vi "Set Drive Motors.vi"(5 "Disable":bool, 6 "Drive PID Slot":i32, 7 "Max Velocity(CP100ms)":dbl=200.0, 8 "Control Mode":T1 items=["PercentOutput"=0, "Position"=1, "Velocity"=2, "Current"=3, "Follower"=5, "MotionProfile"=6, "MotionMagic"=7, "MotionProfileArc"=10, "Disabled"=15], 9 "Motor List":T2[](array[typedef])=[enum."Right-Front", enum."Left-Front", enum."Left-Back", enum."Right-Back"], 10 "Swerve Data":T3 {"Back Right"."Angle" scale format="%.3f"; "Back Right"."Velocity" scale=-1.0..1.0 scale format="%.1f"; "Back Left"."Angle" scale format="%.3f"; "Back Left"."Velocity" scale=-1.0..1.0 scale format="%.1f"; "Front Left"."Angle" scale format="%.3f"; "Front Left"."Velocity" scale=-1.0..1.0 scale format="%.1f"; "Front Right"."Angle" scale format="%.3f"; "Front Right"."Velocity" scale=-1.0..1.0 scale format="%.1f"}, 11 "Drive Refs":T7[](array[typedef])) -> (1 "Speeds":dbl[](array[numeric]), 3 "Array Out":T7[](array[typedef]))   [LabVIEW 2023, in "Thor-SwerveDrive_ACT.lvlib"]
uses:
  Thor-SwerveDrive_ACT.lvlib
  <vilib>/Rock Robotics/WPI/ThirdParty/Phoenix-LabVIEW/Motor Controller/Controls/CTRE_Phoenix_MotorControl_ControlMode.ctl
  <vilib>/Rock Robotics/SystemInterfaces/DIO/FPGA_DIOPWMChannel.ctl
  <vilib>/Rock Robotics/WPI/PWM/WPI_PWMDeadband.ctl
  <vilib>/Rock Robotics/WPI/MotorControl/WPI_MotorControlType.ctl
  <vilib>/Rock Robotics/SystemInterfaces/DIO/FPGA_DIOChannel.ctl
  <vilib>/Rock Robotics/WPI/MotorControl/WPI_MotorControlDeviceRef.ctl
  Shared Code/TypeDefs/Level_Velocity plus-minus 1.ctl
  Shared Code/TypeDefs/Dial_Compase heading unit circle CCW positive.ctl
  Shared Code/TypeDefs/Cluster_Module Velocity-Direction-Rotations.ctl
  Shared Code/TypeDefs/Cluster_Swerve 4 Steer and Velocity.ctl
  Shared Code/TypeDefs/ENUM_Motor Index.ctl
panel:
  # "\"Front\" of Robot"
  # "Right Hand Rule"
  # "X"
  # "+CCW"
  # "Y"
  # "(0,0)"
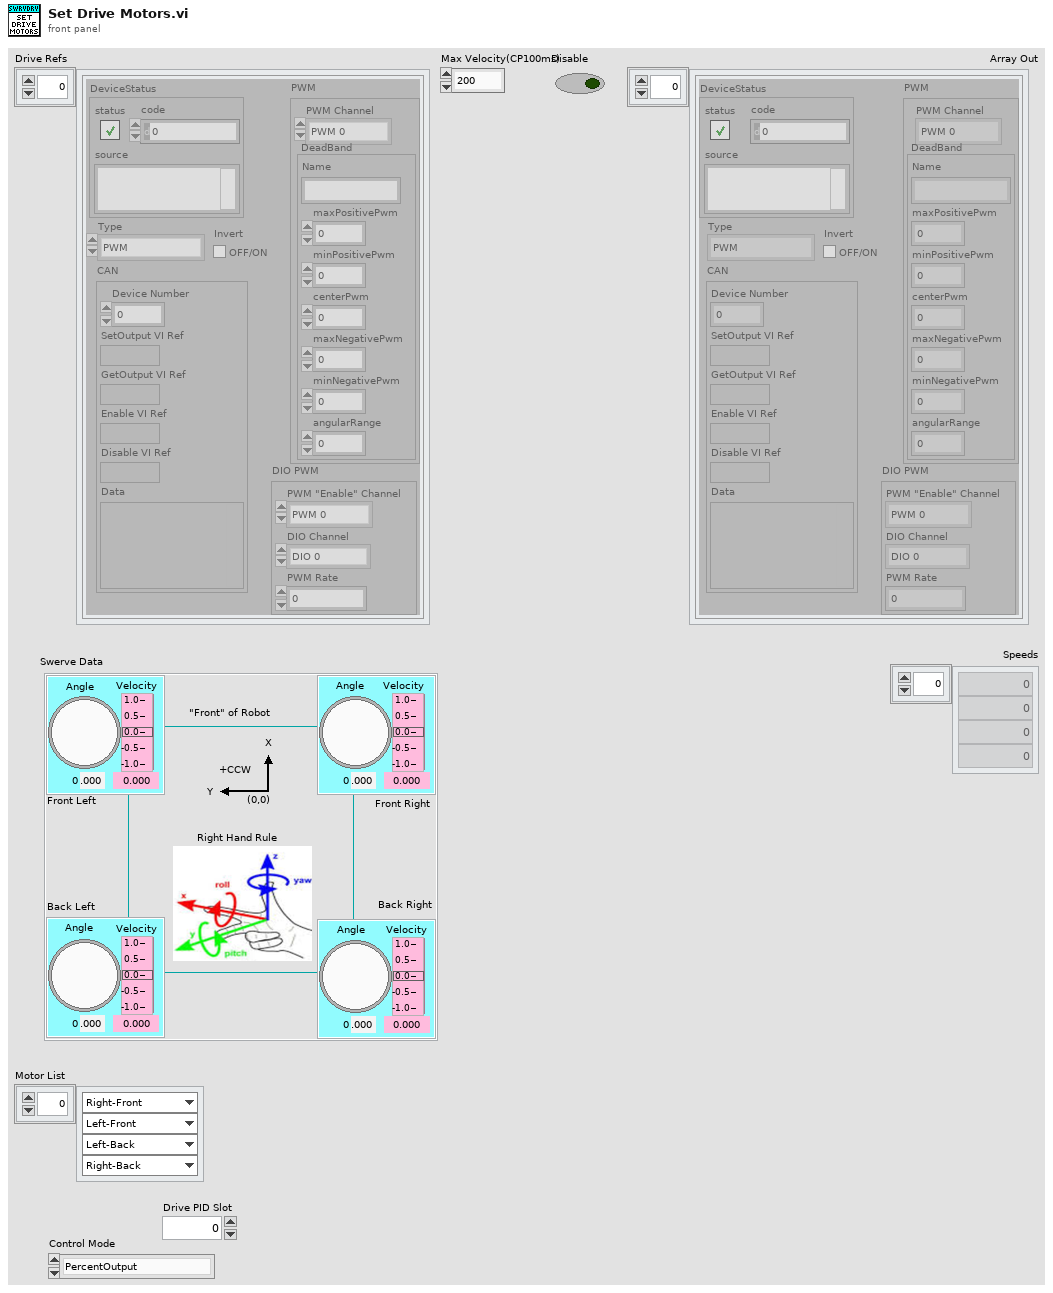
[diagram p1: front panel]
types:
  T1 = typedef "CTRE_Phoenix_MotorControl_ControlMode.ctl" = u16
  T2 = typedef "ENUM_Motor Index.ctl" = enum16{"Left-Front", "Right-Front", "Left-Back", "Right-Back"}
  T3 = typedef "Cluster_Swerve 4 Steer and Velocity.ctl" = cluster{"Front Right":T4, "Front Left":T4, "Back Left":T4, "Back Right":T4}
  T4 = typedef "Cluster_Module Velocity-Direction-Rotations.ctl" = cluster{"Velocity":T5, "Angle":T6, "Rotations Count":dbl}
  T5 = typedef "Level_Velocity plus-minus 1.ctl" = dbl
  T6 = typedef "Dial_Compase heading unit circle CCW positive.ctl" = dbl
  T7 = typedef "WPI_MotorControlDeviceRef.ctl" = cluster{"DeviceStatus":errorcluster, "Type":T8, "PWM":cluster{"PWM Channel":T9, "DeadBand":T10}, "CAN":cluster{"Device Number":u8, "SetOutput VI Ref":variant, "GetOutput VI Ref":variant, "Enable VI Ref":variant, "Disable VI Ref":variant, "Data":variant}, "Invert":bool, "DIO PWM":cluster{"PWM \"Enable\" Channel":T9, "DIOChannel":T11, "PWM Rate":dbl}}
  T8 = typedef "WPI_MotorControlType.ctl" = enum16{"PWM", "CAN", "DIO PWM"}
  T9 = typedef "FPGA_DIOPWMChannel.ctl" = enum8{"PWM 0", "PWM 1", "PWM 2", "PWM 3", "PWM 4", "PWM 5", "PWM 6", "PWM 7", "PWM 8", "PWM 9", "PWM MXP 0", "PWM MXP 1", "PWM MXP 2", "PWM MXP 3", "PWM MXP 4", "PWM MXP 5", "PWM MXP 6", "PWM MXP 7", "PWM MXP 8", "PWM MXP 9", "Invalid"}
  T10 = typedef "WPI_PWMDeadband.ctl" = cluster{"Name":string, "maxPositivePwm":i32, "minPositivePwm":i32, "centerPwm":i32, "maxNegativePwm":i32, "minNegativePwm":i32, "angularRange":u16}
  T11 = typedef "FPGA_DIOChannel.ctl" = enum8{"DIO 0", "DIO 1", "DIO 2", "DIO 3", "DIO 4", "DIO 5", "DIO 6", "DIO 7", "DIO 8", "DIO 9", "DIO MXP 0", "DIO MXP 1", "DIO MXP 2", "DIO MXP 3", "DIO MXP 4", "DIO MXP 5", "DIO MXP 6", "DIO MXP 7", "DIO MXP 8", "DIO MXP 9", "DIO MXP 10", "DIO MXP 11", "DIO MXP 12", "DIO MXP 13", "DIO MXP 14", "DIO MXP 15", "SPI Port CS1", "SPI Port CS2", "SPI Port CS3", "SPI Port MISO", "SPI Port MOSI", "Invalid"}
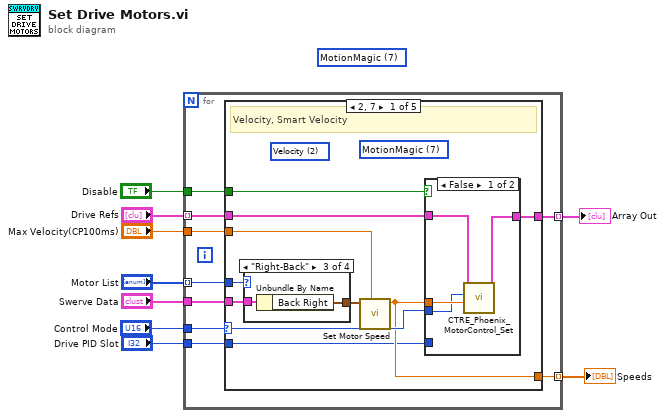
[diagram p0: block diagram]
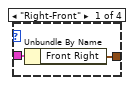
[diagram p3: hidden frame]
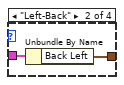
[diagram p4: hidden frame]
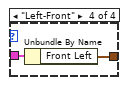
[diagram p5: hidden frame]
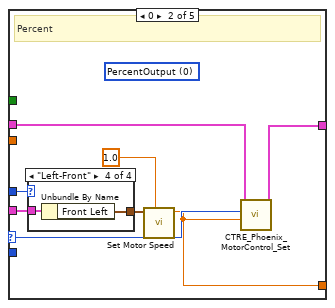
[diagram p6: hidden frame]
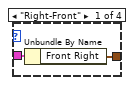
[diagram p7: hidden frame]
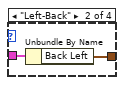
[diagram p8: hidden frame]
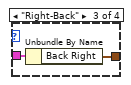
[diagram p9: hidden frame]
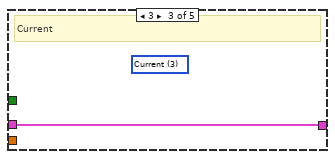
[diagram p10: hidden frame]
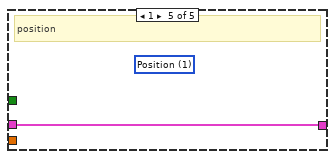
[diagram p12: hidden frame]
diagram:
  (unwired) T1 7 items=["PercentOutput"=0, "Position"=1, "Velocity"=2, "Current"=3, "Follower"=5, "MotionProfile"=6, "MotionMagic"=7, "MotionProfileArc"=10, "Disabled"=15] ("Control Mode")
  n1 = for {
    tunnel: "Drive Refs" -> [w18] mode=indexing
    tunnel: "Control Mode" -> [w17]
    tunnel: "Drive PID Slot" -> [w16]
    tunnel: [w15] -> w9 mode=indexing
    tunnel: "Max Velocity(CP100ms)" -> [w12]
    tunnel: "Motor List" -> [w14] mode=indexing
    tunnel: "Swerve Data" -> [w13]
    tunnel: [w11] -> w3 mode=indexing
    tunnel: "Disable" -> [w10]
    n2 = case shown="2, 7" w17 {
      selector: w17 -> [w27 w48 _ _ _]
      tunnel: w18 -> [w28 w49 w58 w59 w60]
      tunnel: w16 -> [w20 _ _ _ _]
      tunnel: [w26 w47 w58 w59 w60] -> w15
      tunnel: w14 -> [w24 w45 _ _ _]
      tunnel: w13 -> [w25 w46 _ _ _]
      tunnel: w12 -> [w22 _ _ _ _]
      tunnel: [w21 w42 _ _ _] -> w11
      tunnel: w10 -> [w19 _ _ _ _]
      frame 2, 7 {
        (unwired) T1 7 items=["PercentOutput"=0, "Position"=1, "Velocity"=2, "Current"=3, "Follower"=5, "MotionProfile"=6, "MotionMagic"=7, "MotionProfileArc"=10, "Disabled"=15] ("Control Mode")
        (unwired) T1 2 items=["PercentOutput"=0, "Position"=1, "Velocity"=2, "Current"=3, "Follower"=5, "MotionProfile"=6, "MotionMagic"=7, "MotionProfileArc"=10, "Disabled"=15] ("Control Mode")
        # "Velocity, Smart Velocity"
        n3 = case shown="\"Right-Back\"" w24 {
          tunnel: w25 -> [w35 w37 w39 w41]
          tunnel: [w34 w36 w38 w40] -> w23
          frame "Right-Front" {
            n4 = Unbundle By Name(w35) -> ("Front Right"=w34:T4)
          }
          frame "Left-Back" {
            n5 = Unbundle By Name(w37) -> ("Back Left"=w36:T4)
          }
          frame "Right-Back" {
            n6 = Unbundle By Name(w39) -> ("Back Right"=w38:T4)
          }
          frame "Left-Front" {
            n7 = Unbundle By Name(w41) -> ("Front Left"=w40:T4)
          }
        }
        n8 = call "Set Motor Speed.vi"("Max Velocity"=w22, "Front Left"=w23) -> ("Velocity Value Set Out"=w21:dbl)  [unwired: 9 in]
        n9 = case shown="False" w19 {
          tunnel: w28 -> [w32 w33]
          tunnel: w27 -> [w29 _]
          tunnel: [w31 w33] -> w26
          tunnel: w21 -> [w30 _]
          tunnel: w20 -> [_ _]
          frame False {
            n10 = call <vilib>:"CTRE_Phoenix_MotorControl_Set.vi"("Output"=w30, "Control Mode"=w29, "PhoenixMotorControlDevRef"=w32) -> ("PhoenixMotorControlDevRef"=w31:T7)  [unwired: 7 in, 1 out]
          }
          frame True {
          }
        }
      }
      frame 0 {
        (unwired) T1 0 items=["PercentOutput"=0, "Position"=1, "Velocity"=2, "Current"=3, "Follower"=5, "MotionProfile"=6, "MotionMagic"=7, "MotionProfileArc"=10, "Disabled"=15] ("Control Mode")
        # "Percent"
        n11 = case shown="\"Left-Front\"" w45 {
          tunnel: w46 -> [w51 w53 w55 w57]
          tunnel: [w50 w52 w54 w56] -> w44
          frame "Right-Front" {
            n12 = Unbundle By Name(w51) -> ("Front Right"=w50:T4)
          }
          frame "Left-Back" {
            n13 = Unbundle By Name(w53) -> ("Back Left"=w52:T4)
          }
          frame "Right-Back" {
            n14 = Unbundle By Name(w55) -> ("Back Right"=w54:T4)
          }
          frame "Left-Front" {
            n15 = Unbundle By Name(w57) -> ("Front Left"=w56:T4)
          }
        }
        n16 = call "Set Motor Speed.vi"("Max Velocity"=1.0, "Front Left"=w44) -> ("Velocity Value Set Out"=w42:dbl)  [unwired: 9 in]
        n17 = call <vilib>:"CTRE_Phoenix_MotorControl_Set.vi"("Output"=w42, "Control Mode"=w48, "PhoenixMotorControlDevRef"=w49) -> ("PhoenixMotorControlDevRef"=w47:T7)  [unwired: 7 in, 1 out]
      }
      frame 3 {
        (unwired) T1 3 items=["PercentOutput"=0, "Position"=1, "Velocity"=2, "Current"=3, "Follower"=5, "MotionProfile"=6, "MotionMagic"=7, "MotionProfileArc"=10, "Disabled"=15] ("Control Mode")
        # "Current"
      }
      frame Default {
      }
      frame 1 {
        (unwired) T1 1 items=["PercentOutput"=0, "Position"=1, "Velocity"=2, "Current"=3, "Follower"=5, "MotionProfile"=6, "MotionMagic"=7, "MotionProfileArc"=10, "Disabled"=15] ("Control Mode")
        # "position"
      }
    }
  }
  "Array Out" <- w9
  "Speeds" <- w3
